vi "Keithley 6517A Trigger Config.vi"(0 "GPIB address":string="27", 1 "count (set:0)":u16(ring) items=["set  value", "infinite", "min", "max"], 2 "count value":dbl=1.0 min=1.0 max=99999.0 step=1.0, 4 "protocol":bool=TRUE, 5 "direction":bool, 6 "ssync i/o (line 1:0)":u16(ring) items=["line 1", "line 2", "line 3", "line 4", "line 5", "line 6"], 8 "async input (line 2:1)":u16(ring)=1 items=["line 1", "line 2", "line 3", "line 4", "line 5", "line 6"], 9 "delay (secs)":dbl min=0.0 max=999999.999 format="%.3f", 10 "async output (line 1:0)":u16(ring) items=["line 1", "line 2", "line 3", "line 4", "line 5", "line 6"], 11 "error in":T1, 12 "source (imm:1)":u16(ring)=1 items=["hold", "immediate", "timer", "manual", "bus", "trigger link", "external"], 13 "timer value (secs)":dbl=0.001 min=0.001 max=999999.999 format="%.3f") -> (15 "error out":T1)   [LabVIEW 2013]
doc: "This VI is used to configure the settings for the Measure Layer (Trigger) of the trigger model. The model consists of 3 layers, the Arm Layer, the Scan Layer (Arm2), and the Measure Layer (Trigger).\n\nIn general, measure events control the measurement (or scan) rate."
panel:
  # "source\nacceptor"
  # "asynchronous\nsemi-synchronous"
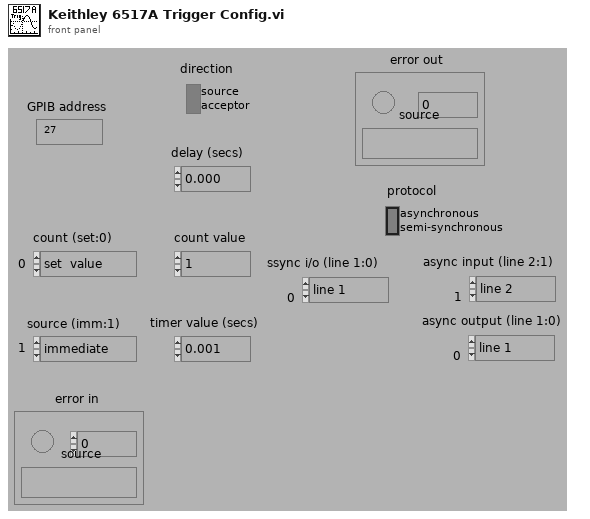
[diagram p1: front panel]
types:
  T1 = cluster{"error":bool, "code":i32, "source":string}
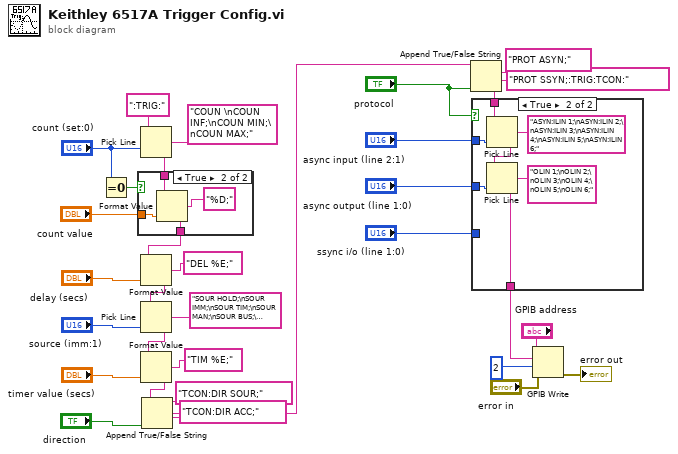
[diagram p0: block diagram]
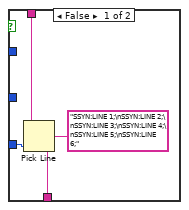
[diagram p2: hidden frame]
diagram:
  n1 = Equal To 0?(x="count (set:0)") -> (x = 0?=w27:bool)
  n2 = Pick Line(string ("")=":TRIG:", multi-line string="COUN \nCOUN INF;\nCOUN MIN;\nCOUN MAX;", line index="count (set:0)") -> (output string=w28:string)
  n3 = case shown="True" w27 {
    tunnel: "count value" -> [_ w37]
    tunnel: w28 -> [w33 w36]
    tunnel: [w33 w34] -> w19
    frame False {
    }
    frame True {
      n4 = Format Value(string ("")=w36, format string="%D;", value (0)=w37) -> (output string=w34:string)
    }
  }
  n5 = Format Value(string ("")=w19, format string="DEL %E;", value (0)="delay (secs)") -> (output string=w18:string)
  n6 = Pick Line(string ("")=w18, multi-line string="SOUR HOLD;\nSOUR IMM;\nSOUR TIM;\nSOUR MAN;\nSOUR BUS;\nSOUR TLIN;\nSOUR EXT;", line index="source (imm:1)") -> (output string=w15:string)
  n7 = Format Value(string ("")=w15, format string="TIM %E;", value (0)="timer value (secs)") -> (output string=w14:string)
  n8 = Append True/False String(1:"direction", 2:"TCON:DIR ACC;", 3:"TCON:DIR SOUR;", 4:w14) -> (0:w13:string)
  n9 = Append True/False String(1:"protocol", 2:"PROT SSYN;:TRIG:TCON:", 3:"PROT ASYN;", 4:w13) -> (0:w9:string)
  n10 = case shown="True" "protocol" {
    tunnel: w9 -> [w39 w45]
    tunnel: "async input (line 2:1)" -> [_ w44]
    tunnel: "async output (line 1:0)" -> [_ w43]
    tunnel: [w38 w42] -> w3
    tunnel: "ssync i/o (line 1:0)" -> [w40 _]
    frame False {
      n11 = Pick Line(string ("")=w39, multi-line string="SSYN:LINE 1;\nSSYN:LINE 2;\nSSYN:LINE 3;\nSSYN:LINE 4;\nSSYN:LINE 5;\nSSYN:LINE 6;", line index=w40) -> (output string=w38:string)
    }
    frame True {
      n12 = Pick Line(string ("")=w45, multi-line string="ASYN:ILIN 1;\nASYN:ILIN 2;\nASYN:ILIN 3;\nASYN:ILIN 4;\nASYN:ILIN 5;\nASYN:ILIN 6;", line index=w44) -> (output string=w47:string)
      n13 = Pick Line(string ("")=w47, multi-line string="OLIN 1;\nOLIN 2;\nOLIN 3;\nOLIN 4;\nOLIN 5;\nOLIN 6;", line index=w43) -> (output string=w42:string)
    }
  }
  n14 = GPIB Write(0:"GPIB address", 1:w3, 2:2, 3:"error in") -> (6:→"error out":errorcluster)  [unwired: 1 in, 1 out]
